vi "PH_Timing.evt call set Phase FEs.vi"(0 "i ref in":refnum<vi>, 2 "Instance":string, 3 "Phase FEs":T1 {"Phase" format="%#_12p"}, 5 "error in (no error)":errorcluster) -> (14 "i ref out":refnum<vi>, 19 "error out":errorcluster)   [LabVIEW 2014, in "PH_Timing.lvlib"]
doc: "This VI calls the case \"PhaseFEs\" by a simple call."
uses:
  PH_Timing.lvlib
  PH_Timing.Phase FEs.ctl
  CS_Core/CSSystem/CoreLib/CoreLib.double 2 byte array.vi
  CS_Core/BaseProcess/BaseProcess.lvlib
  CS_Core/CSSystem/CoreLib/CoreLib.lvlib
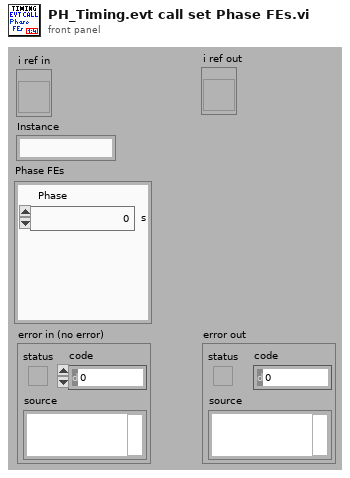
[diagram p1: front panel]
types:
  T1 = typedef "PH_Timing.lvlib/PH_Timing.Phase FEs.ctl" = cluster{"Phase":dbl}
  T2 = typedef "CoreDefs.rawDataType.ctl" = i8[]
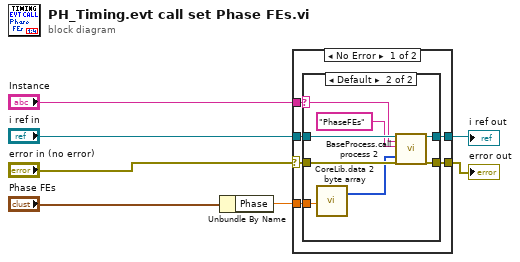
[diagram p0: block diagram]
diagram:
  n1 = Unbundle By Name("Phase FEs") -> ("Phase"=w1:dbl)
  n2 = case shown="No Error" "error in (no error)" {
    selector: "error in (no error)" -> [w9 w24]
    tunnel: [w13 w25] -> w4
    tunnel: [w12 w24] -> w3
    tunnel: "i ref in" -> [w11 w25]
    tunnel: "Instance" -> [w10 _]
    tunnel: w1 -> [w8 _]
    frame No Error {
      n3 = case shown="Default" w10 {
        selector: w10 -> [_ w18]
        tunnel: [w15 w23] -> w13
        tunnel: [w14 w22] -> w12
        tunnel: w11 -> [w15 w21]
        tunnel: w9 -> [w14 w20]
        tunnel: w8 -> [_ w17]
        frame "N/A" {
        }
        frame Default {
          n4 = call-poly "CoreLib.data 2 byte array.vi"("f64"=w17) -> ("byteArray out"=w16:T2)  [unwired: 18 in]
          n5 = call "BaseProcess.call process 2.vi"("i ref in"=w21, "Object"=w18, "Selector"="PhaseFEs", "Data"=w16, "error in (no error)"=w20) -> ("i ref out"=w23:refnum<vi>, "error out"=w22:errorcluster)  [unwired: 13 in]
        }
      }
    }
    frame Error {
    }
  }
  "error out" <- w3
  "i ref out" <- w4
